vi "Set Call Status.vi"(8 "error in":errorcluster, 9 "Details":string, 10 "Status Code":T2=enum."INTERNAL", 11 "gRPCid in":T1) -> (0 "error out":errorcluster, 3 "gRPCid out":T1)   [LabVIEW 2019, in "grpc-lvsupport.lvlib"]
uses:
  grpc-lvsupport.lvlib
  gRPC Status Code.ctl
  grpcId.ctl
  <vilib>/Utility/error.llb/Error Cluster From Error Code.vi
  <resource>/labview_grpc_server.dll
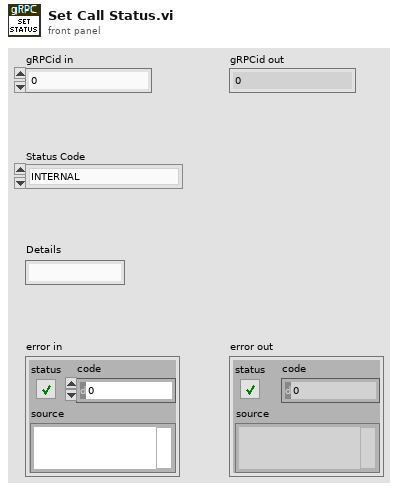
[diagram p1: front panel]
types:
  T1 = typedef "grpc-lvsupport.lvlib/grpcId.ctl" = u64
  T2 = typedef "grpc-lvsupport.lvlib/gRPC Status Code.ctl" = enum16{"OK", "CANCELLED", "UNKNOWN", "INVALID_ARGUMENT", "DEADLINE_EXCEEDED", "NOT_FOUND", "ALREADY_EXISTS", "PERMISSION_DENIED", "RESOURCE_EXHAUSTED", "FAILED_PRECONDITION", "ABORTED", "OUT_OF_RANGE", "UNIMPLEMENTED", "INTERNAL", "UNAVAILABLE", "DATA_LOSS", "UNAUTHENTICATED"}
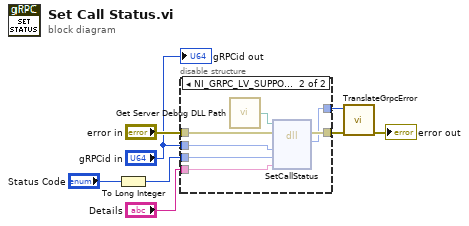
[diagram p0: block diagram]
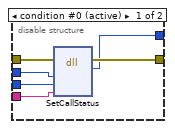
[diagram p2: hidden frame]
diagram:
  n1 = To Long Integer(number="Status Code") -> (32bit integer=w2:i32)
  n2 = disable-structure shown="NI_GRPC_LV_SUPPORT_DEBUG==True&&RUN_TIME_ENGINE==False" {
    disable-tunnel: "error in" -> [w14 w21]
    disable-tunnel: [w13 w20] -> w7
    disable-tunnel: "gRPCid in" -> [w12 w19]
    disable-tunnel: [w11 w17] -> w6
    disable-tunnel: "Details" -> [w10 w16]
    disable-tunnel: w2 -> [w9 w15]
    frame condition #0 (active) {
      n3 = dll-call lib="C:/Program Files (x86)/National Instruments/LabVIEW 2024/resource/labview_grpc_server.*" fn="SetCallStatus"(error in=w14, "grpcId"=w12, "errorCode"=w9, "errorMessage"=w10) -> (error out=w13:errorcluster, "return type"=w11:i32)  [unwired: 5 in, 1 out]
    }
    frame condition #1 {
      n4 = call "Get Server Debug DLL Path.vi"() -> ("DLL Path"=w18:path)
      n5 = dll-call lib="?" fn="SetCallStatus"(path in=w18, error in=w21, "grpcId"=w19, "errorCode"=w15, "errorMessage"=w16) -> (error out=w20:errorcluster, "return type"=w17:i32)  [unwired: 4 in, 1 out]
    }
  }
  n6 = call "TranslateGrpcError.vi"("error in"=w7, "Error Code"=w6) -> ("error out"=→"error out":errorcluster)  [unwired: 9 in]
  "gRPCid out" <- "gRPCid in"
